vi "Drive Controller.vi"(8 "error in":errorcluster) -> ()   [LabVIEW 2016]
doc: "This VI executes continuously carrying out the current operation and responding to updates or new operation requests. It will often contain the timing or control code that is difficult to place directly in TeleOp. This VI generally opens all sensors and motors and isolates the rest of the robot code from knowing implementation details of how the operations are carried out."
uses:
  Drive Setpoints.ctl
  Drive Operations.ctl
  <vilib>/Rock Robotics/WPI/SafetyOutput/WPI_SafetyOutputConfigMenu.ctl
  <vilib>/Rock Robotics/WPI/Utilities/WPI_GetSetVariantRefNum.vi
panel:
  out "Setpoints":T1(graph)
  out "Current\nCmd":string
  # "Tip: It may be helpful to observe inputs and sensor values.\nYou may also want to display tuning or debugging controls."
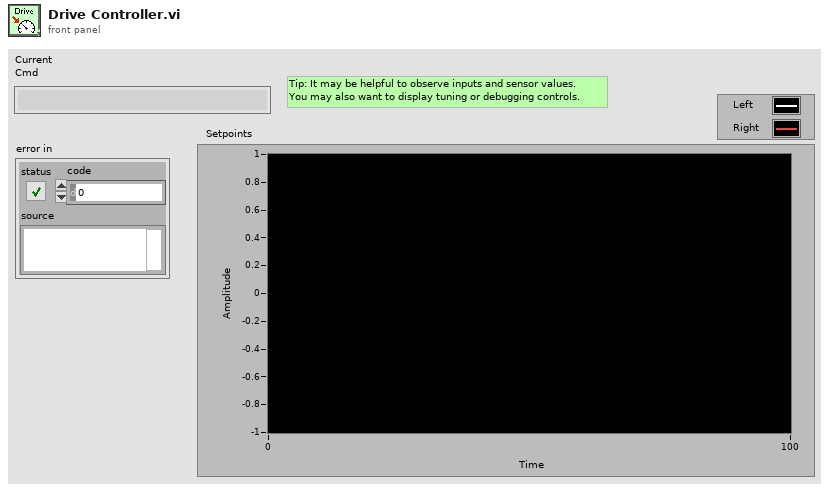
[diagram p1: front panel]
types:
  T1 = cluster{"Left Setpoint":dbl, "Right Setpoint":dbl}
  T2 = typedef "WPI_SafetyOutputConfigMenu.ctl" = enum16{"Enable", "Disable"}
  T3 = typedef "Drive Setpoints.ctl" = cluster{"Operation":T4, "Left Setpoint":dbl, "Right Setpoint":dbl, "Duration":dbl}
  T4 = typedef "Drive Operations.ctl" = enum16{"Reserve", "Read Current", "Immediate", "Drive for Time", "Drive for Distance"}
  T5 = typedef "WPI_RobotDriveDevRef.ctl" = cluster{"DevStatus":errorcluster, "Motors[]":T6[], "Square Inputs":bool, "Max Output":dbl}
  T6 = typedef "WPI_MotorControlDeviceRef.ctl" = cluster{"DeviceStatus":errorcluster, "Type":T7, "PWM":cluster{"PWM Channel":T8, "DeadBand":T9}, "CAN":cluster{"Device Number":u8, "SetOutput VI Ref":variant, "GetOutput VI Ref":variant, "Enable VI Ref":variant, "Disable VI Ref":variant, "Data":variant}, "Invert":bool}
  T7 = typedef "WPI_MotorControlType.ctl" = enum16{"PWM", "CAN"}
  T8 = typedef "FPGA_DIOPWMChannel.ctl" = enum8{"PWM 0", "PWM 1", "PWM 2", "PWM 3", "PWM 4", "PWM 5", "PWM 6", "PWM 7", "PWM 8", "PWM 9", "PWM MXP 0", "PWM MXP 1", "PWM MXP 2", "PWM MXP 3", "PWM MXP 4", "PWM MXP 5", "PWM MXP 6", "PWM MXP 7", "PWM MXP 8", "PWM MXP 9", "Invalid"}
  T9 = typedef "WPI_PWMDeadband.ctl" = cluster{"Name":string, "maxPositivePwm":i32, "minPositivePwm":i32, "centerPwm":i32, "maxNegativePwm":i32, "minNegativePwm":i32, "angularRange":u16}
  T10 = typedef "Command Status Info.ctl" = cluster{"Name":string, "Status":T11, "notifier out":T12}
  T11 = typedef "Completion Status.ctl" = enum16{"Successful", "Aborted", "Incomplete"}
  T12 = typedef "Completion Notifier.ctl" = refnum<notifier>
  T13 = cluster{"SubSystem Data":T3, cluster{"Start Time (ms)":u32, "Iterations":i32}, cluster{"Command Info":T10, "Description":string, "SubSystem Data":T3, "notifier out":refnum<notifier>, "Subsystem Name":string}}
  T14 = cluster{"SubSystem Data":T3, cluster{"Start Time (ms)":u32, "Iterations":i32}, "Default Command Arguments":cluster{"Command Info":T10, "Description":string, "SubSystem Data":T3, "notifier out":refnum<notifier>, "Subsystem Name":string}}
  T15 = cluster{"Don't move motors while reserved":dbl, "Don't move motors while reserved":dbl}
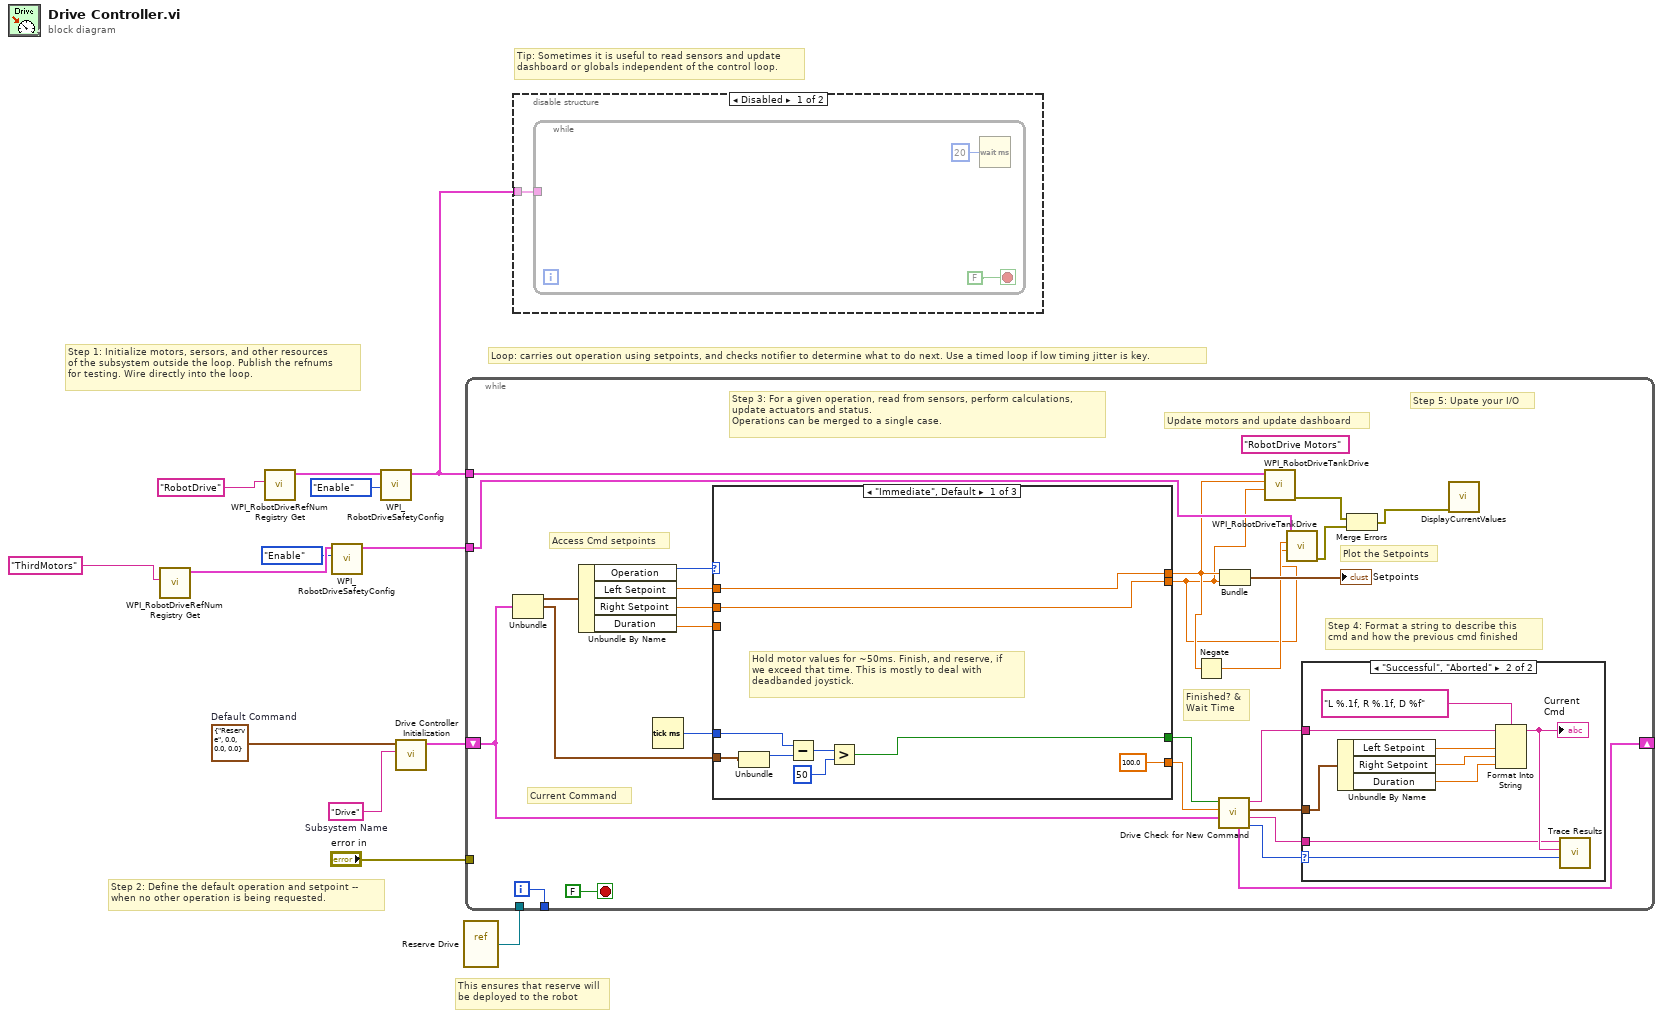
[diagram p0: block diagram]
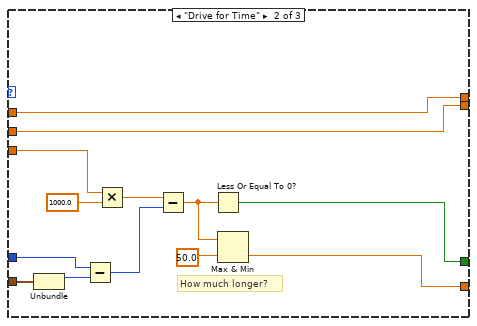
[diagram p4: hidden frame]
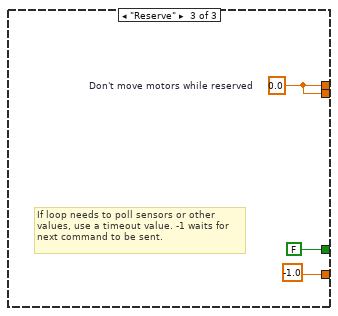
[diagram p5: hidden frame]
diagram:
  w12 = T3 {"Operation"=enum."Reserve", "Left Setpoint"=0.0, "Right Setpoint"=0.0, "Duration"=0.0}  # Default Command
  w13 = "Drive"  # Subsystem Name
  # "This ensures that reserve will\nbe deployed to the robot"
  # "Tip: Sometimes it is useful to read sensors and update\ndashboard or globals independent of the control loop."
  # "Step 2: Define the default operation and setpoint --\nwhen no other operation is being requested."
  # "Step 1: Initialize motors, sersors, and other resources\nof the subsystem outside the loop. Publish the refnums\nfor testing. Wire directly into the loop."
  # "Loop: carries out operation using setpoints, and checks notifier to determine what to do next. Use a timed loop if low timing jitter is key."
  n1 = call <vilib>:"WPI_RobotDriveRefNum Registry Get.vi"("refnum name"="ThirdMotors") -> ("RobotDriveDevRef"=w3:T5)  [unwired: 9 in, 1 out]
  n2 = call <vilib>:"WPI_RobotDriveRefNum Registry Get.vi"("refnum name"="RobotDrive") -> ("RobotDriveDevRef"=w10:T5)  [unwired: 9 in, 1 out]
  n3 = call <vilib>:"WPI_RobotDriveSafetyConfig.vi"("mode"=WPI_SafetyOutputConfigMenu."Enable", "RobotDriveDevRef"=w3) -> ("RobotDriveDevRef"=w2:T5)  [unwired: 8 in, 1 out]
  n4 = call <vilib>:"WPI_RobotDriveSafetyConfig.vi"("mode"=WPI_SafetyOutputConfigMenu."Enable", "RobotDriveDevRef"=w10) -> ("RobotDriveDevRef"=w8:T5)  [unwired: 8 in, 1 out]
  n5 = call "Drive Controller Initialization.vi"("Subsystem Name"=w13, "Default Command"=w12) -> ("output cluster"=w6:T13)  [unwired: 9 in]
  n6 = vi-ref "Reserve Drive.vi"() -> (w5:refnum<vi>)
  n7 = while {
    shift-right: [w28] -> _
    shift-left: w6 -> [w21]
    tunnel: [w38] -> _
    tunnel: w8 -> [w36]
    tunnel: "error in" -> [_]
    tunnel: w5 -> [_]
    tunnel: w2 -> [w20]
    i -> [w38]
    stop <- FALSE stop-if-true
    (unwired) "RobotDrive Motors" ("Name")
    # "Step 5: Upate your I/O"
    # "Step 4: Format a string to describe this\ncmd and how the previous cmd finished"
    # "Current Command"
    # "Update motors and update dashboard"
    # "Plot the Setpoints"
    # "Access Cmd setpoints"
    # "Finished? &\nWait Time"
    # "Step 3: For a given operation, read from sensors, perform calculations,\nupdate actuators and status.\nOperations can be merged to a single case."
    n8 = Unbundle(w21) -> ("SubSystem Data"=w35:T3, w22:cluster{"Start Time (ms)":u32, "Iterations":i32})  [unwired: 1 out]
    n9 = Unbundle By Name(w35) -> ("Operation"=w34:T4, "Left Setpoint"=w33:dbl, "Right Setpoint"=w32:dbl, "Duration"=w31:dbl)
    n10 = Tick Count (ms)() -> (millisecond timer value=w30:u32)
    n11 = case shown="\"Immediate\", Default" w34 {
      tunnel: [100.0 w58 -1.0] -> w27
      tunnel: [w50 w65 FALSE ("ignore previous (F)")] -> w26
      tunnel: w22 -> [w49 w67 _]
      tunnel: [w56 w64 w71] -> w16
      tunnel: [w55 w63 w71] -> w14
      tunnel: w33 -> [w56 w64 _]
      tunnel: w32 -> [w55 w63 _]
      tunnel: w31 -> [_ w62 _]
      tunnel: w30 -> [w51 w61 _]
      frame "Immediate", Default {
        # "Hold motor values for ~50ms. Finish, and reserve, if\nwe exceed that time. This is mostly to deal with\ndeadbanded joystick."
        n12 = Unbundle(w49) -> ("Start Time (ms)"=w52:u32)  [unwired: 1 out]
        n13 = Subtract(x=w51, y=w52) -> (x-y=w53:u32)
        n14 = Greater?(x=w53, y=u8 50 ("Left Motor")) -> (0:w50:bool)
      }
      frame "Drive for Time" {
        # "How much longer?"
        n15 = Unbundle(w67) -> ("Start Time (ms)"=w66:u32)  [unwired: 1 out]
        n16 = Subtract(x=w61, y=w66) -> (x-y=w70:u32)
        n17 = Multiply(x=w62, y=1000.0) -> (x*y=w69:dbl)
        n18 = Subtract(x=w69, y=w70) -> (x-y=w60:dbl)
        n19 = Less Or Equal To 0?(x=w60) -> (x <= 0?=w65:bool)
        n20 = Max & Min(x=w60, y=50.0) -> (min(x,y)=w58:dbl)  [unwired: 1 out]
      }
      frame "Reserve" {
        w71 = 0.0  # Don't move motors while reserved
        # "If loop needs to poll sensors or other\nvalues, use a timeout value. -1 waits for\nnext command to be sent."
      }
    }
    n21 = Negate(x=w16) -> (-x=w15:dbl)
    n22 = call "Drive Check for New Command.vi"("input cluster"=w21, "Wait time (ms)"=w27, "Finished?"=w26) -> ("Completion"=w29:T11, "Subsystem Name"=w23:string, "SetPoint"=w24:T3, "Initial Trace String"=w25:string, "output cluster"=w28:T14)  [unwired: 4 in]
    n23 = Bundle("Don't move motors while reserved"=w16, "Don't move motors while reserved"=w14) -> (→"Setpoints":T15)  [unwired: 1 in]
    n24 = call <vilib>:"WPI_RobotDriveTankDrive.vi"("Right axis value"=w14, "Left axis value"=w16, "RobotDriveDevRef"=w36) -> ("error out"=w18:errorcluster)  [unwired: 6 in, 2 out]
    n25 = call <vilib>:"WPI_RobotDriveTankDrive.vi"("Right axis value"=w14, "Left axis value"=w15, "RobotDriveDevRef"=w20) -> ("error out"=w17:errorcluster)  [unwired: 6 in, 2 out]
    n26 = case shown="\"Successful\", \"Aborted\"" w29 {
      selector: w29 -> [_ w48]
      tunnel: w25 -> [_ w43]
      tunnel: w24 -> [_ w44]
      tunnel: w23 -> [_ w40]
      frame "Incomplete", Default {
        # "Continuing current command"
      }
      frame "Successful", "Aborted" {
        # "Report and setup for next command"
        n27 = Unbundle By Name(w44) -> ("Left Setpoint"=w46:dbl, "Right Setpoint"=w47:dbl, "Duration"=w41:dbl)
        n28 = Format Into String(format string="L %.1f, R %.1f, D %f", initial string=w43, w46, w47, w41) -> (resulting string=w42:string)  [unwired: 1 in, 1 out]
        "Current\nCmd" <- w42
        n29 = call <vilib>:"Trace Results.vi"("Status of previous command"=w48, "Description"=w42, "Subsystem"=w40) -> ()  [unwired: 9 in]
      }
    }
    n30 = Merge Errors(w18, w17) -> (w19:errorcluster)
    n31 = call "DisplayCurrentValues.vi"("error in (no error)"=w19) -> ()  [unwired: 6 in, 5 out]
  }
  n32 = disable-structure shown="Disabled" {
    disable-tunnel: w8 -> [w74 _]
    frame Disabled {
      n33 = while {
        tunnel: w74 -> [_]
        stop <- FALSE stop-if-true
        n34 = Wait (ms)(milliseconds to wait=u32 20) -> ()  [unwired: 1 out]
      }
    }
    frame Enabled {
    }
  }
